vi "Set Address.vi"(8 "error in (no error)":errorcluster, 10 "address":u8, 11 "RRG in":refnum<class "PL Eltochpribor RRG.lvclass">) -> (0 "error out":errorcluster, 3 "RRG out":refnum<class "PL Eltochpribor RRG.lvclass">)   [LabVIEW 2015, in "PL Eltochpribor RRG.lvclass"]
doc: "Sets communication address."
uses:
  PL Eltochpribor RRG.lvclass
  <vilib>/plasmapper/PL Modbus Client/PL Modbus Client.lvclass
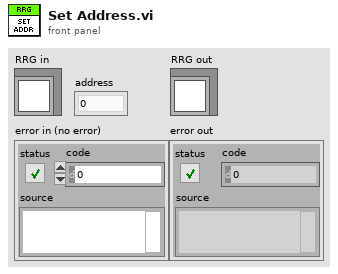
[diagram p1: front panel]
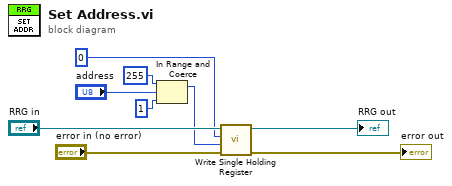
[diagram p0: block diagram]
diagram:
  n1 = In Range and Coerce(upper limit=u8 255, x="address", lower limit=u8 1) -> (coerced(x)=w3:u8)  [unwired: 1 out]
  n2 = call <vilib>:"Write Single Holding Register.vi"("error in (no error)"="error in (no error)", "value"=w3, "address"=u16 0, "MODBUS in"="RRG in") -> ("error out"=→"error out":errorcluster, "MODBUS out"=→"RRG out":refnum<class "PL Eltochpribor RRG.lvclass">)  [unwired: 6 in]
